vi "Example Instrument.Read Configuration File.vi"(8 "error in (no error)":errorcluster, 11 "Example Instrument in":refnum<class "Example Instrument.lvclass">) -> (0 "error out":errorcluster, 3 "Example Instrument out":refnum<class "Example Instrument.lvclass">)   [LabVIEW 2016, in "Example Instrument.lvclass"]
uses:
  Example Instrument.lvclass
  C:/user/patrick/hg/levylab_inst del/lvsrc/SMOs/Instrument/Instrument.lvclass
  Example Instrument.lvclass/Example Instrument.ctl
  Instrument/Instrument.lvclass/Instrument.ctl
  Configuration/Configuration.lvclass
  Instrument/Instrument.lvclass
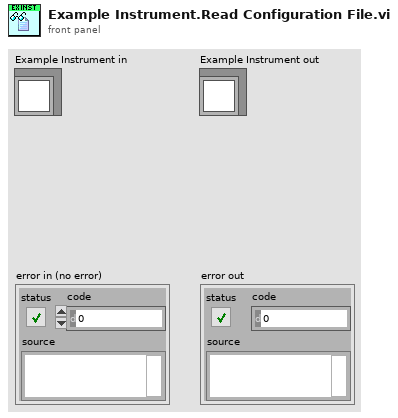
[diagram p1: front panel]
types:
  T1 = typedef "Example Instrument.lvclass/Configuration--Cluster.ctl" = cluster{"Example Setting 1":dbl, "Example Setting 2":dbl, "Example Setting 3":string}
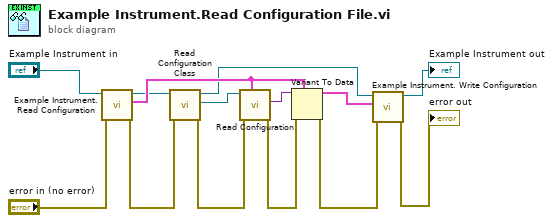
[diagram p0: block diagram]
diagram:
  n1 = call "Example Instrument. Read Configuration.vi"("error in (no error)"="error in (no error)", "Example Instrument in"="Example Instrument in") -> ("error out"=w6:errorcluster, "Ex Configuration"=w10:T1, "Example Instrument out"=w8:refnum<class "Example Instrument.lvclass">)  [unwired: 7 in]
  n2 = call "Read Configuration Class.vi"("error in (no error)"=w6, "Instrument in"=w8) -> ("error out"=w5:errorcluster, "Configuration.lvclass"=w9:refnum<class "Configuration.lvclass">, "Instrument out"=w7:refnum<class "Example Instrument.lvclass">)  [unwired: 7 in]
  n3 = call "Read Configuration.vi"("INI Fomatted Cluster Type"=w10, "error in (no error)"=w5, "Configuration in"=w9) -> ("error out"=w13:errorcluster, "Configuration"=w14:variant)  [unwired: 6 in, 1 out]
  n4 = Variant To Data(error in=w13, type=w10, Variant=w14) -> (data=w12:T1, error out=w11:errorcluster)
  n5 = call "Example Instrument. Write Configuration.vi"("error in (no error)"=w11, "Configuration"=w12, "Example Instrument in"=w7) -> ("error out"=→"error out":errorcluster, "Example Instrument out"=→"Example Instrument out":refnum<class "Example Instrument.lvclass">)  [unwired: 7 in]
